vi "niRFUtil TRC Save Traces to File (Multiple Traces, 2D).vi"(0 "File Path In (dialog if empty)":T2, 1 "Append to File? (new file:F)":bool, 5 "Measurement Traces":T1 format="%.2f", 7 "Format (%.12f)":T4="%.12f", 9 "Delimiter (\\t)":T3="\t", 11 "error in":errorcluster, 12 "Transpose? (no:F)":bool) -> (15 "error out":errorcluster)   [LabVIEW 2015, in "niRFUtil.lvlib"]
uses:
  niRFUtil.lvlib
  Includes/niRFUtil INC File Path.ctl
  Includes/niRFUtil INC Text File Format Specifier.ctl
  Includes/niRFUtil INC Text File Delimiter.ctl
  Includes/niRFUtil INC Trace Array.ctl
panel:
  out "File Path Out":T2
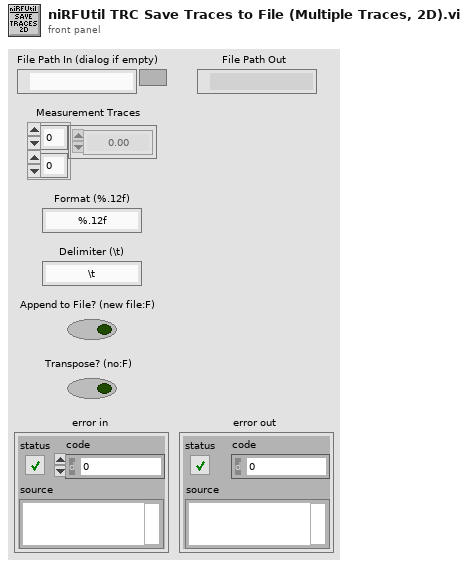
[diagram p1: front panel]
types:
  T1 = typedef "niRFUtil.lvlib/niRFUtil INC Trace Array.ctl" = dbl[][]
  T2 = typedef "niRFUtil.lvlib/niRFUtil INC File Path.ctl" = path
  T3 = typedef "niRFUtil.lvlib/niRFUtil INC Text File Delimiter.ctl" = string
  T4 = typedef "niRFUtil.lvlib/niRFUtil INC Text File Format Specifier.ctl" = string
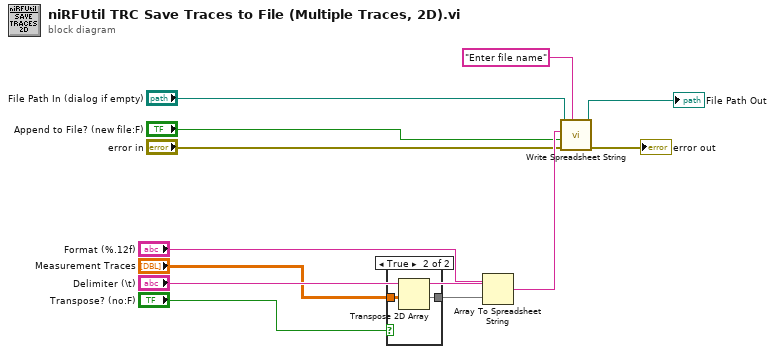
[diagram p0: block diagram]
diagram:
  n1 = case shown="True" "Transpose? (no:F)" {
    tunnel: [w13 w15] -> w12
    tunnel: "Measurement Traces" -> [w13 w14]
    frame False {
    }
    frame True {
      n2 = Transpose 2D Array(2D array=w14) -> (transposed array=w15:T1)
    }
  }
  n3 = Array To Spreadsheet String(delimiter (Tab)="Delimiter (\\t)", array=w12, 3:"Format (%.12f)") -> (spreadsheet string=w10:string)
  n4 = call <vilib>:"Write Spreadsheet String.vi"("prompt"="Enter file name", "error in"="error in", "append to file? (new file:F)"="Append to File? (new file:F)", "spreadsheet string"=w10, "file path (dialog if empty)"="File Path In (dialog if empty)") -> ("error out"=→"error out":errorcluster, "path"=→"File Path Out":path)  [unwired: 2 in, 3 out]
